vi "X Axis Speed Conversion sub_VI.vi"(11 "Speed (m/s)":dbl) -> (3 "PWM Duty %":dbl)   [LabVIEW 2017]
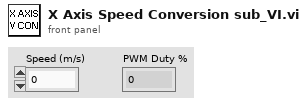
[diagram p1: front panel]
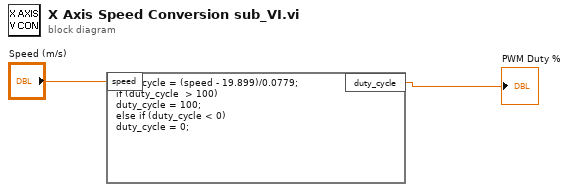
[diagram p0: block diagram]
diagram:
  n1 = formula code="duty_cycle = (speed - 19.899)/0.0779;\nif (duty_cycle  > 100)\nduty_cycle = 100;\nelse if (duty_cycle < 0)\nduty_cycle = 0;"("speed"="Speed (m/s)") -> ("duty_cycle"=→"PWM Duty %":dbl)
